vi "VI_BSA.vi"() -> ()   [LabVIEW 2019]
uses:
  <vilib>/Analysis/2dsp.llb/Real FFT.vi
  <vilib>/Analysis/NI_AALPro.lvlib
panel:
  out "Zeitsignal 4":dynamicdata(graph) caption="Sawtooth"
  out "Zeitsignal 3":dynamicdata(graph) caption="Sawtooth"
  out "Zeitsignal 2":dynamicdata(graph) caption="Sawtooth"
  out "Zeitsignal 1":dynamicdata(graph) caption="Sawtooth"
  out "Amplitude":dbl[](graph)
  out "Phase":dbl[](graph)
  out "Sawtooth":dynamicdata(graph)
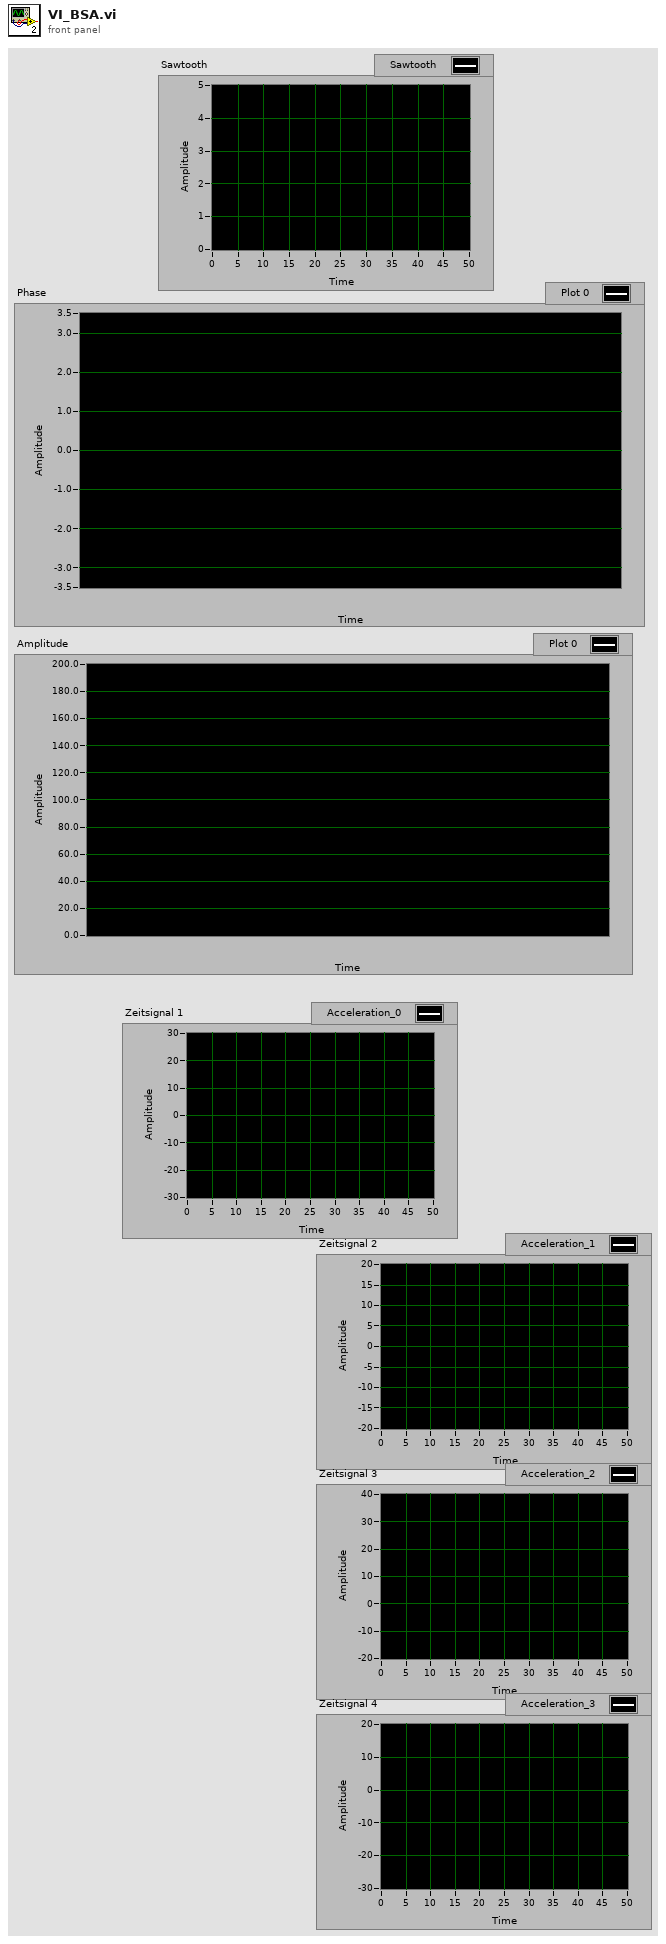
[diagram p1: front panel]
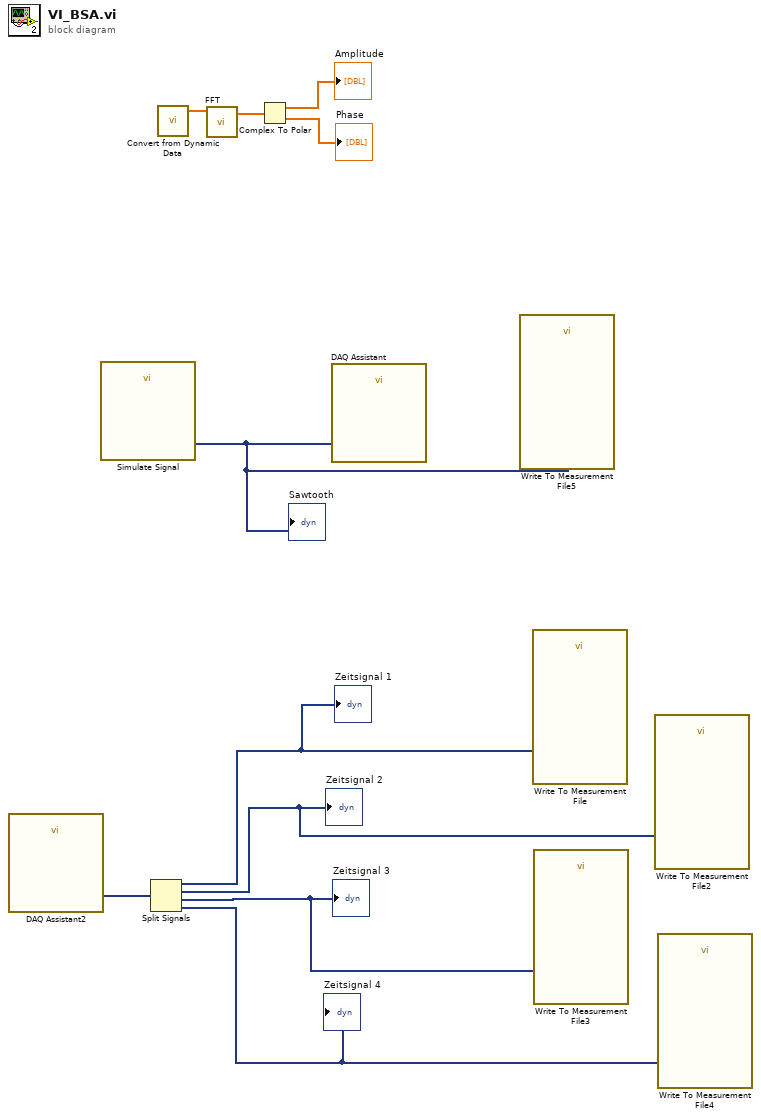
[diagram p0: block diagram]
diagram:
  n1 = call "DAQ Assistant2"() -> ("data"=w6:dynamicdata)  [unwired: 17 in, 2 out]
  n2 = call "Simulate Signal"() -> ("Sawtooth"=w1:dynamicdata)  [unwired: 14 in, 1 out]
  "Sawtooth" <- w1
  n3 = Split Signals(w6) -> (w5:dynamicdata, w4:dynamicdata, w3:dynamicdata, w2:dynamicdata)  [unwired: 4 in]
  "Zeitsignal 1" <- w5
  "Zeitsignal 2" <- w4
  "Zeitsignal 3" <- w3
  "Zeitsignal 4" <- w2
  n4 = call "Convert from Dynamic Data"() -> ("Array"=w7:dbl[])  [unwired: 4 in]
  n5 = call-poly <vilib>:"FFT.vi"("X"=w7) -> ("FFT {X}"=w10:cdb[])  [unwired: 9 in, 1 out]
  n6 = Complex To Polar(r * e^(i*theta)=w10) -> (r=→"Amplitude":dbl[], theta=→"Phase":dbl[])
  n7 = call "DAQ Assistant"("data"=w1) -> ()  [unwired: 17 in, 2 out]
  n8 = call "Write To Measurement File5"("Signals"=w1) -> ()  [unwired: 16 in, 3 out]
  n9 = call "Write To Measurement File"("Signals"=w5) -> ()  [unwired: 16 in, 3 out]
  n10 = call "Write To Measurement File3"("Signals"=w3) -> ()  [unwired: 16 in, 3 out]
  n11 = call "Write To Measurement File2"("Signals"=w4) -> ()  [unwired: 16 in, 3 out]
  n12 = call "Write To Measurement File4"("Signals"=w2) -> ()  [unwired: 16 in, 3 out]
